vi "OA Get String.vi"(7 "uiStringLen":u32, 9 "pcStringValue":string, 10 "pcModeParam":string, 11 "pcModeName":string) -> (1 "pcStringValue out":string, 3 "function return":u32)   [LabVIEW 2018, in "Copy of Andor SDK.lvlib"]
doc: "EXPNETTYPE unsigned int WINAPI OA_GetString(const char * const pcModeName, const char * const pcModeParam, char * pcStringValue, const unsigned int uiStringLen);"
uses:
  Copy of Andor SDK.lvlib
  <userlib>/Andor SDK/ATMCD32D.dll
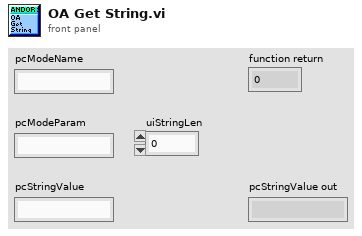
[diagram p1: front panel]
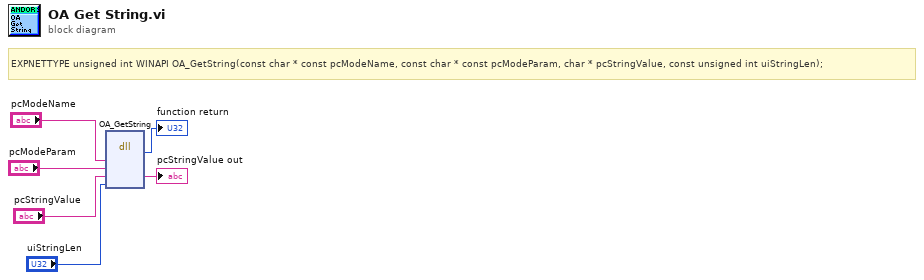
[diagram p0: block diagram]
diagram:
  # "EXPNETTYPE unsigned int WINAPI OA_GetString(const char * const pcModeName, const char * const pcModeParam, char * pcStringValue, const unsigned int uiStringLen);"
  n1 = dll-call lib="C:/Program Files (x86)/National Instruments/LabVIEW 2018/user.lib/Andor SDK/ATMCD32D.*" fn="OA_GetString"("pcModeName"="pcModeName", "pcModeParam"="pcModeParam", "pcStringValue"="pcStringValue", "uiStringLen"="uiStringLen") -> (→"function return":u32, "pcStringValue"=→"pcStringValue out":string)  [unwired: 6 in, 2 out]
